vi "Host - FoE From Bitfile.vi"(8 "error in (no error)":errorcluster, 10 "Firmware filename":path, 11 "Slave Ref in":refnum<k21>) -> (0 "error out":errorcluster, 1 "File Byte Array":u8[](array[numeric]), 2 "Firmware filename out":path, 3 "Slave Ref out":refnum<k21>, 5 "Need Reset":bool)   [LabVIEW 2016, in "Scan Engine Custom Device.lvlib"]
uses:
  Scan Engine Custom Device.lvlib
  <resource>/objmgr/IndComECAT.rc
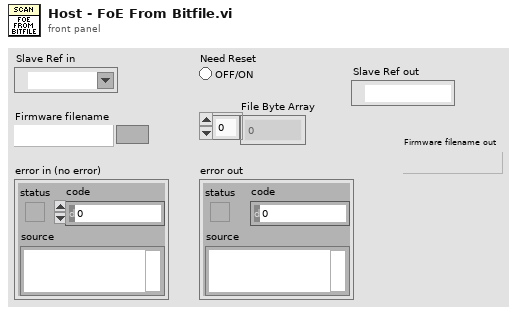
[diagram p1: front panel]
types:
  T1 = enum16{"open", "replace", "create", "open or create", "replace or create", "replace or create with confirmation"}
  T2 = typedef "niFpgaBitfileStructure.ctl" = cluster{"Bitfile":T3, "VI":T4, "Project":T11}
  T3 = typedef "niFpgaBitfileStructure_Bitfile.ctl" = cluster{"SignatureRegister":u8[], "SignatureGuids":u8[], "SignatureNames":u8[], "SignatureBitstream":u8[], "TimeStamp":string, "CompileStatus":string, "BitstreamVersion":u32}
  T4 = typedef "niFpgaBitfileStructure_VI.ctl" = cluster{"Name":string, "RegisterMap":T5[], "Icon":T10}
  T5 = typedef "nirviControlStructure.ctl" = cluster{"Name":string, "Hidden":bool, "Indicator":bool, "Flattened Type":string, "Grouping":cluster{"Grouped":bool, "Member Names":string[], "Member IDs":u32[]}, "Address":u32, "Size":u32, "Class":u32, "Internal":bool, "Typedef":T6, "ID":u32, "Bidirectional":bool, "Synchronous":bool, "Mechanical Action":T7, "Sub Controls":T8[], "Access May Timeout":bool, "Register Node":bool}
  T6 = typedef "nirviTypdefDescription.ctl" = cluster{"Typedef":bool, "Path":path}
  T7 = typedef "nirviMechanicalAction.ctl" = enum8{"Switch When Pressed", "Switch When Released", "Switch Until Released", "Latch When Pressed", "Latch When Released", "Latch Until Released"}
  T8 = typedef "nirviSubControlStructure.ctl" = cluster{"Name":string, "flattened Type":string, "Cluster Information":T9, "Typedef":T6}
  T9 = typedef "nirviClusterElementControl.ctl" = cluster{"Name Hierarchy":string[], "Item Order":u32[]}
  T10 = typedef "imagedata.ctl" = cluster{"image type":i32, "image depth":i32, "image":u8[], "mask":u8[], "colors":u32[], "Rectangle":cluster{"left":i16, "top":i16, "right":i16, "bottom":i16}}
  T11 = typedef "niFpgaBitfileStructure_Project.ctl" = cluster{"TargetClass":string, "AutoRunWhenDownloaded":bool, "CompilationResults":string, "MultipleUserClocks":bool, "AllowEnableRemoval":bool}
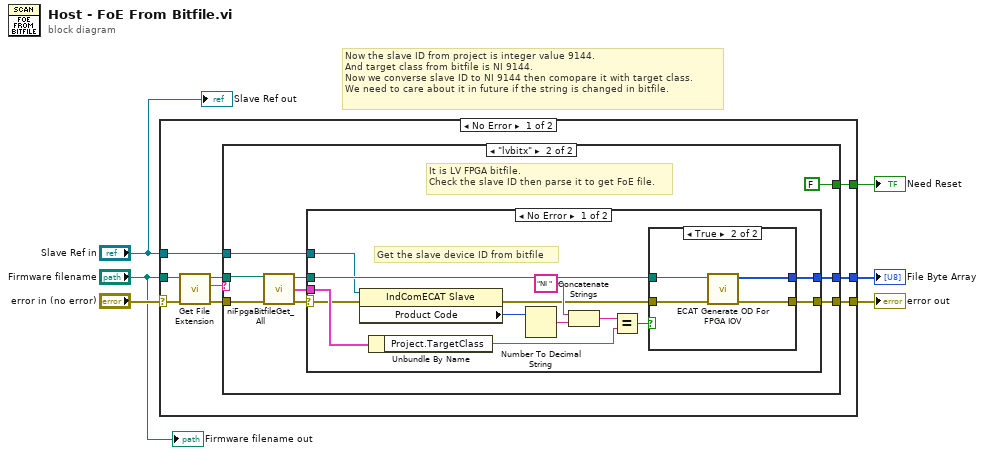
[diagram p0: block diagram]
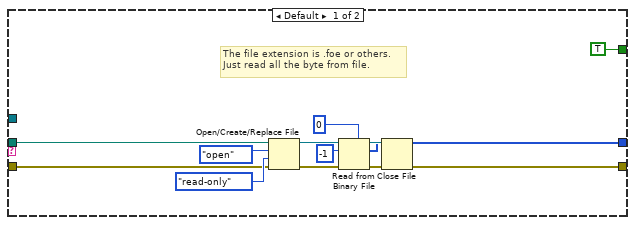
[diagram p2: hidden frame]
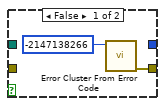
[diagram p3: hidden frame]
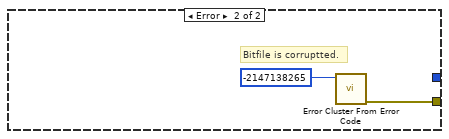
[diagram p4: hidden frame]
diagram:
  # "Now the slave ID from project is integer value 9144.\nAnd target class from bitfile is NI 9144.\nNow we converse slave ID to NI 9144 then comopare it with target class.\nWe need to care about it in future if the string is changed in bitfile."
  n1 = case shown="No Error" "error in (no error)" {
    selector: "error in (no error)" -> [w10 w58]
    tunnel: "Firmware filename" -> [w11 _]
    tunnel: "Slave Ref in" -> [w15 _]
    tunnel: [w14 w58] -> w6
    tunnel: [w8 _] -> w5
    tunnel: [w7 _] -> w4
    frame No Error {
      n2 = call <vilib>:"Get File Extension.vi"("error in (no error)"=w10, "file"=w11) -> ("error out"=w12:errorcluster, "lowercase file extension"=w9:string, "dup file"=w13:path)  [unwired: 7 out]
      n3 = case shown="\"lvbitx\"" w9 {
        tunnel: w15 -> [_ w32]
        tunnel: [w19 w34] -> w14
        tunnel: w13 -> [w17 w35]
        tunnel: w12 -> [w26 w36]
        tunnel: [w18 w30] -> w8
        tunnel: [TRUE FALSE] -> w7
        frame Default {
          # "The file extension is .foe or others. \nJust read all the byte from file."
          n4 = Open/Create/Replace File(file path (use dialog)=w17, error in=w26, operation (0:open)=T1."open", access (0:read/write)=enum16{"read/write", "read-only", "write-only"}."read-only") -> (refnum out=w24:refnum<file>, error out=w25:errorcluster)  [unwired: 2 in, 1 out]
          n5 = Read from Binary File(5:u8 0, 8:w25, 10:-1 ("count (1)"), 11:w24) -> (0:w21:errorcluster, 2:w18:u8[], 3:w20:refnum<file>)  [unwired: 2 in, 1 out]
          n6 = Close File(refnum=w20, error in=w21) -> (error out=w19:errorcluster)  [unwired: 1 out]
        }
        frame "lvbitx" {
          # "It is LV FPGA bitfile. \nCheck the slave ID then parse it to get FoE file."
          n7 = call <vilib>:"niFpgaBitfileGet_All.vi"("bitfile path"=w35, "error in (no error)"=w36) -> ("bitfile structure"=w33:T2, "error out"=w31:errorcluster)  [unwired: 11 in, 1 out]
          n8 = case shown="No Error" w31 {
            selector: w31 -> [w39 _]
            tunnel: w35 -> [w48 _]
            tunnel: [w47 w56] -> w34
            tunnel: [w43 _] -> w30
            tunnel: w33 -> [w42 _]
            tunnel: w32 -> [w40 _]
            frame No Error {
              # "Get the slave device ID from bitfile"
              n9 = property class="IndComECAT Slave"(reference=w40, error in=w39) -> (error out=w37:errorcluster, "Product Code"=w38:u32)  [unwired: 1 out]
              n10 = Unbundle By Name(w42) -> ("Project.TargetClass"=w41:string)
              n11 = Number To Decimal String(number=w38) -> (decimal integer string=w46:string)  [unwired: 1 in]
              n12 = Concatenate Strings("NI " ("string"), w46) -> (w44:string)
              n13 = Equal?(x=w44, y=w41) -> (x = y?=w49:bool)
              n14 = case shown="True" w49 {
                tunnel: w48 -> [_ w54]
                tunnel: w37 -> [_ w55]
                tunnel: [w51 w53] -> w47
                tunnel: [_ w52] -> w43
                frame False {
                  n15 = call <vilib>:"Error Cluster From Error Code.vi"("error code (0)"=-2147138266) -> ("error out"=w51:errorcluster)  [unwired: 8 in]
                }
                frame True {
                  n16 = call "ECAT Generate OD For FPGA IOV.vi"("error in"=w55, "Input bitfile path"=w54) -> ("error out"=w53:errorcluster, "File Byte Array"=w52:u8[])  [unwired: 6 in, 2 out]
                }
              }
            }
            frame Error {
              # "Bitfile is corruptted."
              n17 = call <vilib>:"Error Cluster From Error Code.vi"("error code (0)"=-2147138265) -> ("error out"=w56:errorcluster)  [unwired: 8 in]
            }
          }
        }
      }
    }
    frame Error {
    }
  }
  "error out" <- w6
  "File Byte Array" <- w5
  "Need Reset" <- w4
  "Slave Ref out" <- "Slave Ref in"
  "Firmware filename out" <- "Firmware filename"
